vi "Python Email.vi"(0 "Path to Python.exe":path=path "C:/Users/zstreeter/AppData/Local/Programs/Python/Python35-32/python.exe", 5 "Script Path":path=path "C:/Users/zstreeter/Documents/Projects/TI sbRIO/Source/Email Handler/gmail_script.py", 7 "To:":string, 9 "Subject:":string, 11 "Message:":string) -> (4 "Raw Python String Output":string="successfully sent the mail\r\n", 6 "Converted Output":i32, 8 "Return Code":i32, 10 "Standard Error":string, 15 "error out":errorcluster)   [LabVIEW 2019]
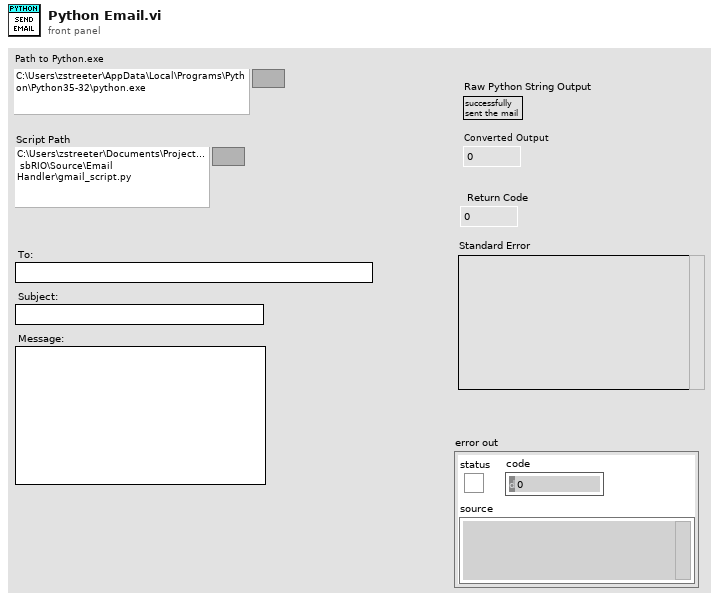
[diagram p1: front panel]
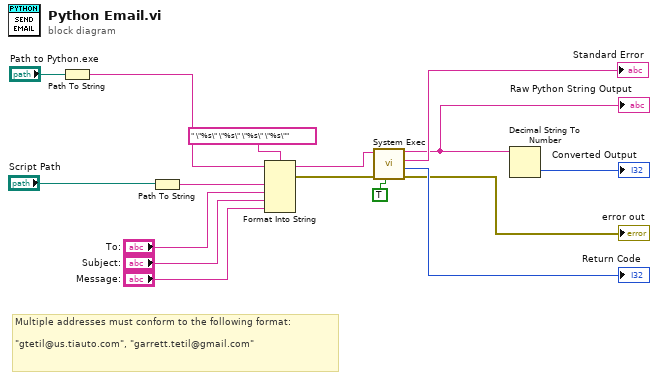
[diagram p0: block diagram]
diagram:
  # "Multiple addresses must conform to the following format:\n\n\"gtetil@us.tiauto.com\", \"garrett.tetil@gmail.com\""
  n1 = Path To String(path="Path to Python.exe") -> (string=w9:string)
  n2 = Path To String(path="Script Path") -> (string=w13:string)
  n3 = Format Into String(format string=" \"%s\" \"%s\" \"%s\" \"%s\"", initial string=w9, w13, "To:", "Subject:", "Message:") -> (resulting string=w12:string, error out=w10:errorcluster)  [unwired: 1 in]
  n4 = call <vilib>:"System Exec.vi"("run minimized? (F)"=TRUE, "error in (no error)"=w10, "command line"=w12) -> ("error out"=→"error out":errorcluster, "return code"=→"Return Code":i32, "standard error"=→"Standard Error":string, "standard output"=w7:string)  [unwired: 5 in]
  "Raw Python String Output" <- w7
  n5 = Decimal String To Number(string=w7) -> (number=→"Converted Output":i32)  [unwired: 2 in, 1 out]
